vi "Pretrigger Buffer New vers.vi"(5 "Mode":enum16{"Initialize", "Add", "Read"}(ring), 7 "Pretrigger Length":i32, 8 "# Channels":i32, 10 "New Data":sgl[](array[numeric])) -> (2 "Pretrigger Data":sgl[][](array[numeric]))   [LabVIEW 2019]
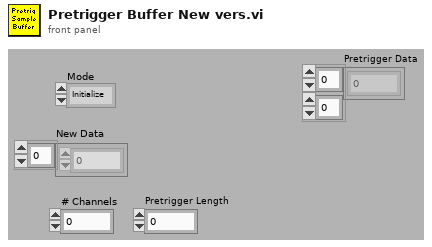
[diagram p1: front panel]
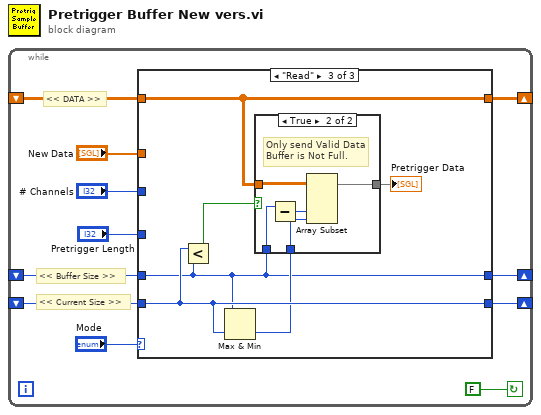
[diagram p0: block diagram]
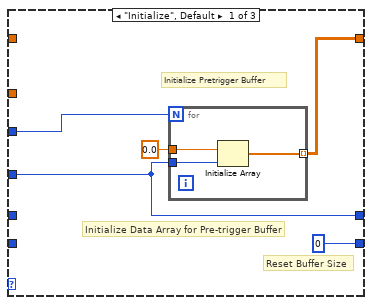
[diagram p2: hidden frame]
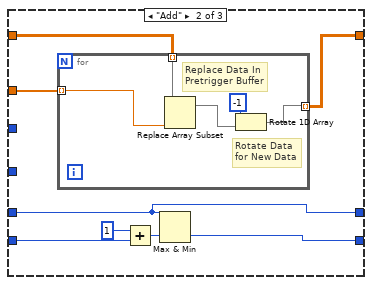
[diagram p3: hidden frame]
diagram:
  n1 = while {
    shift-right: [w5] -> _
    shift-left: _ -> [w10]
    shift-right: [w7] -> _
    shift-left: _ -> [w2]
    shift-right: [w4] -> _
    shift-left: _ -> [w3]
    stop <- FALSE continue-if-true
    # "<< Buffer Size >>"
    # "<< Current Size >>"
    # "<< DATA >>"
    n2 = case shown="\"Read\"" "Mode" {
      tunnel: w10 -> [_ w27 w37]
      tunnel: "# Channels" -> [w15 _ _]
      tunnel: "New Data" -> [_ w25 _]
      tunnel: [0 w21 w35] -> w7
      tunnel: "Pretrigger Length" -> [w13 _ _]
      tunnel: [w12 w26 w37] -> w5
      tunnel: [w13 w22 w33] -> w4
      tunnel: w3 -> [_ w22 w33]
      tunnel: w2 -> [_ w23 w35]
      frame "Initialize", Default {
        # "Reset Buffer Size"
        # "Initialize Pretrigger Buffer"
        # "Initialize Data Array for Pre-trigger Buffer"
        n3 = for {
          N: w15 -> [_]
          tunnel: sgl 0.0 ("element") -> [w19]
          tunnel: w13 -> [w18]
          tunnel: [w17] -> w12 mode=indexing
          n4 = Initialize Array(w19, w18) -> (w17:sgl[])
        }
      }
      frame "Add" {
        n5 = for {
          tunnel: w27 -> [w32] mode=indexing
          tunnel: [w30] -> w26 mode=indexing
          tunnel: w25 -> [w29] mode=indexing
          # "Rotate Data\nfor New Data"
          # "Replace Data In \nPretrigger Buffer"
          n6 = Replace Array Subset(array=w32, new element=w29) -> (w31:sgl[])  [unwired: 1 in]
          n7 = Rotate 1D Array(1:w31, 2:-1 ("n")) -> (0:w30:sgl[])
        }
        n8 = Add(x=1, y=w23) -> (x+y=w24:i32)
        n9 = Max & Min(x=w22, y=w24) -> (min(x,y)=w21:i32)  [unwired: 1 out]
      }
      frame "Read" {
        n10 = Less?(x=w35, y=w33) -> (x < y?=w38:bool)
        n11 = Max & Min(x=w33, y=w35) -> (min(x,y)=w34:i32)  [unwired: 1 out]
        n12 = case shown="True" w38 {
          tunnel: w37 -> [w39 w44]
          tunnel: [w39 w43] -> w36
          tunnel: w34 -> [_ w41]
          tunnel: w33 -> [_ w40]
          frame False {
            # "Pretrigger is full"
          }
          frame True {
            # "Only send Valid Data\nBuffer is Not Full."
            n13 = Subtract(x=w40, y=w41) -> (x-y=w42:i32)
            n14 = Array Subset(array=w44, index (col)=w42, length (col)=w41) -> (w43:sgl[][])  [unwired: 2 in]
          }
        }
        "Pretrigger Data" <- w36
      }
    }
  }
